vi "I2C Stop.vi"(8 "error in (no error)":errorcluster, 11 "I2C Task In":T1) -> (0 "error out":errorcluster, 3 "I2C Task Out":T1)   [LabVIEW 2017, in "I2C.lvlib"]
doc: "Sends a stop bit to the slave device according to the I2C specifications."
uses:
  <vilib>/robotics/Protocols/I2C/DAQmx/I2C.lvlib
  <vilib>/robotics/Protocols/I2C/DAQmx/Private/I2C Tasks.ctl
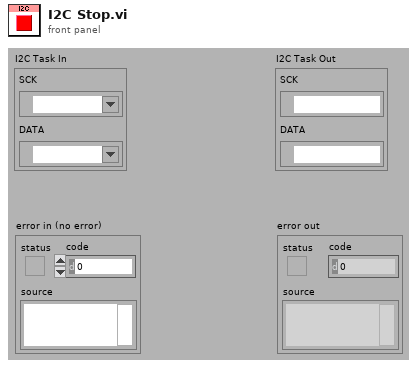
[diagram p1: front panel]
types:
  T1 = typedef "I2C.lvlib/I2C Tasks.ctl" = cluster{"SCK":refnum<k21>, "DATA":refnum<k21>}
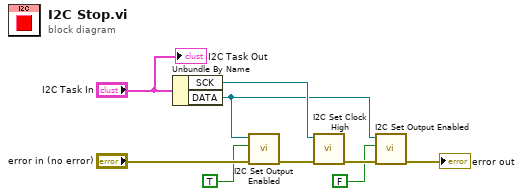
[diagram p0: block diagram]
diagram:
  n1 = Unbundle By Name("I2C Task In") -> ("SCK"=w6:refnum<k21>, "DATA"=w4:refnum<k21>)
  n2 = call <vilib>:"I2C Set Output Enabled.vi"("error in (no error)"="error in (no error)", "Output Enabled (T:Enable)"=TRUE, "Task In"=w4) -> ("error out"=w7:errorcluster)  [unwired: 7 in, 1 out]
  n3 = call <vilib>:"I2C Set Clock High.vi"("error in (no error)"=w7, "Task In"=w6) -> ("error out"=w5:errorcluster)  [unwired: 8 in, 1 out]
  n4 = call <vilib>:"I2C Set Output Enabled.vi"("error in (no error)"=w5, "Output Enabled (T:Enable)"=FALSE, "Task In"=w4) -> ("error out"=→"error out":errorcluster)  [unwired: 7 in, 1 out]
  "I2C Task Out" <- "I2C Task In"
